vi "DSDLL Digitizing Process.vi"(8 "error in":errorcluster, 11 "dsdll session":variant) -> (0 "error out":errorcluster, 3 "auxiliary data out":variant)   [LabVIEW 2020, in "DSDLL Virtual Digitizer.lvlib"]
doc: "This is called assynchronously! It is process where niScope digitizers digitize samples, then fetching them and returning them via queue to the calling process. It handles both single shot and continuous sampling. For single shot sampling it returns the data in blocks of predifined size after all sampling is done. For streaming mode it streams the data blocks continuously. In any case the calling process must take the data from queue in parallel with this VI otherwise it will overflow! The function also returnes status in the data packet which may be used to determine progess of the digitizing and state of the memory buffer.\nThis VI also returns auxiliary data, i.e. structure with scaling factors, time stamps and measured temperature during sampling."
uses:
  DSDLL Virtual Digitizer.lvlib
  DSDLL Session.ctl
  dsdll/dsdll_instance.ctl
  dsdll/dsdll_device_record.ctl
  DSDLL Process Config.ctl
  DSDLL Data Packet.ctl
  DSDLL Aux Record Data.ctl
  dsdll/dsdll_capture_wave_auto_float32.vi
  dsdll/dsdll.lvlib
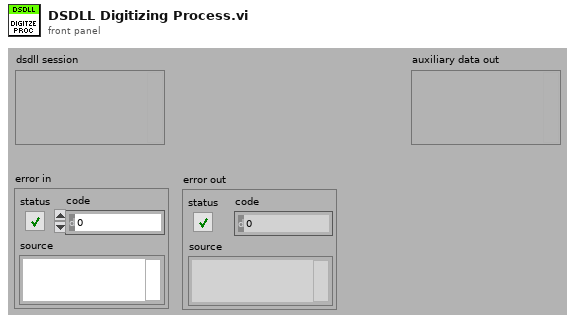
[diagram p1: front panel]
types:
  T1 = typedef "DSDLL Virtual Digitizer.lvlib/DSDLL Session.ctl" = cluster{"dsdll":T2, "channels":i32, "device id":i32, "channel idns":string[], "proc setup":T4, "samples count":i32, "fs [Hz]":dbl}
  T2 = typedef "dsdll.lvlib/dsdll_instance.ctl" = cluster{"dsdll path":path, "dsdll handle":u8[], "output devices":T3[], "capture devices":T3[]}
  T3 = typedef "dsdll.lvlib/dsdll_device_record.ctl" = cluster{"guid":u8[], "name":string}
  T4 = typedef "DSDLL Virtual Digitizer.lvlib/DSDLL Process Config.ctl" = cluster{"packet size [smpl]":i32, "current timeout [s]":dbl, "blk2blk timeout [s]":dbl, "event time":timestamp, "data queue":refnum<queue>, "stop notifier":refnum<notifier>, "proc ref":refnum<vi>}
  T5 = typedef "DSDLL Virtual Digitizer.lvlib/DSDLL Aux Record Data.ctl" = cluster{"time stamp [s]":dbl[], "gain":dbl[], "increment [s]":dbl, "valid?":bool, "abs timestamp":timestamp}
  T6 = typedef "DSDLL Virtual Digitizer.lvlib/DSDLL Data Packet.ctl" = cluster{"int32":i32[][], "card buffer [%]":dbl, "all done?":bool, "offset [smpl]":i32, "sampling?":bool, "queue buffer [%]":dbl, "count [smpl]":i32, "valid?":bool}
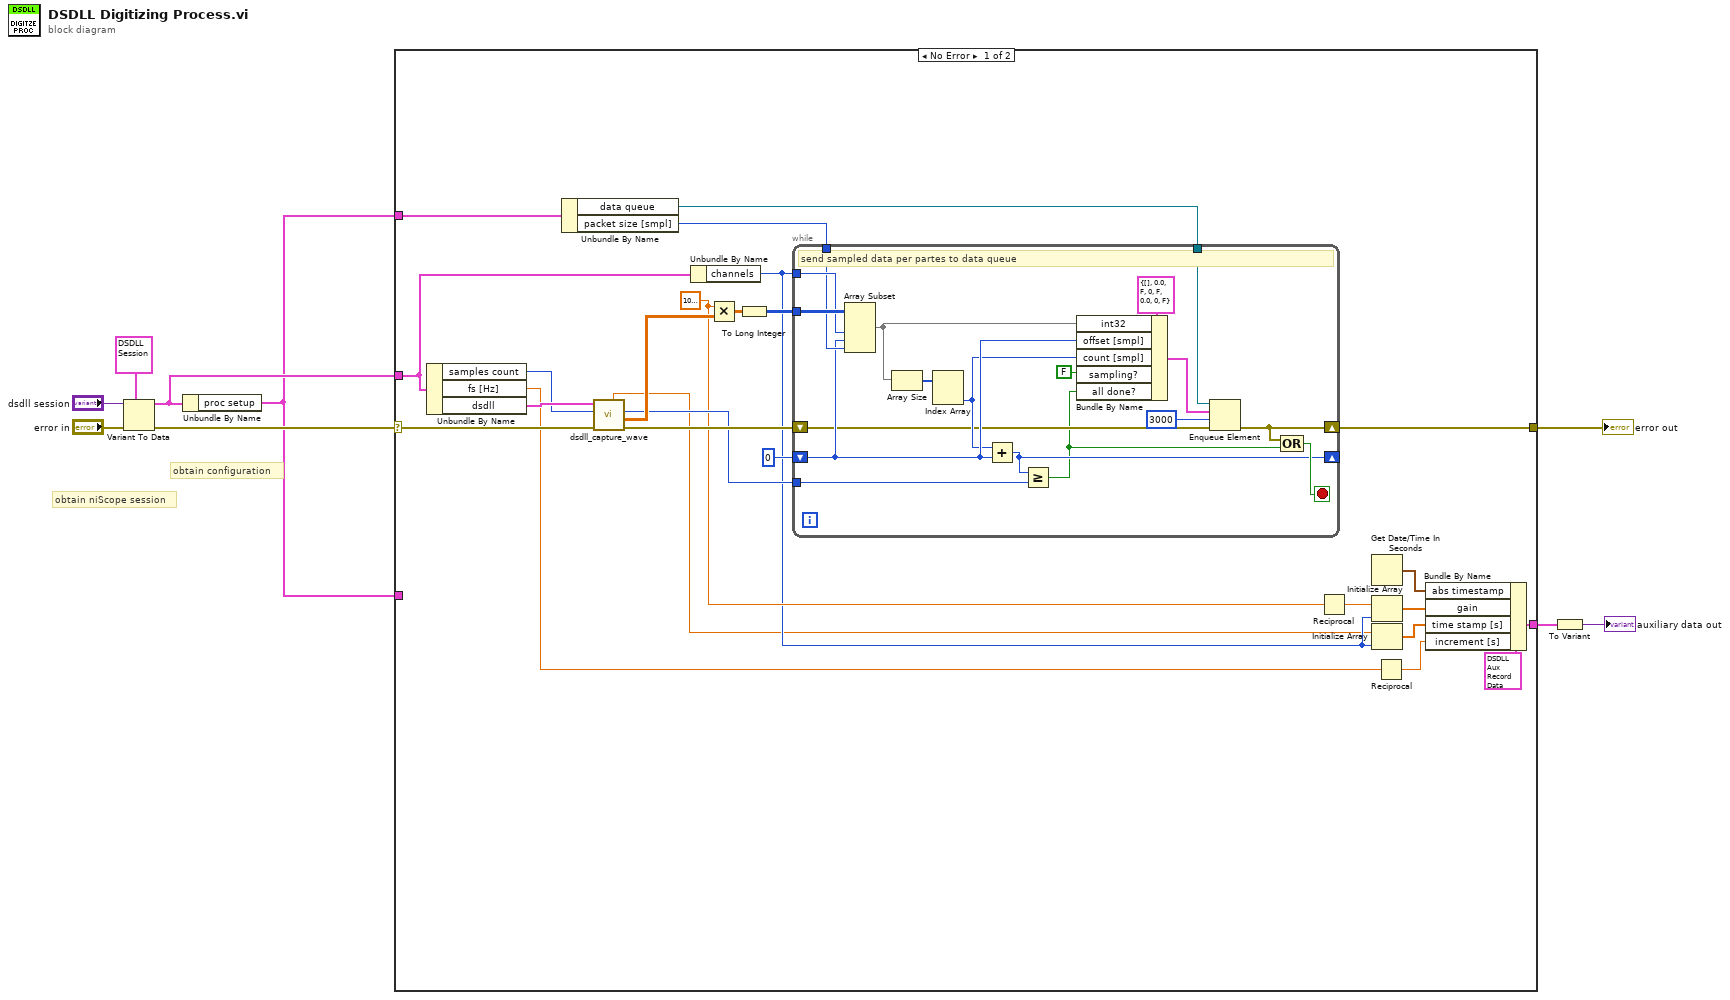
[diagram p0: block diagram]
diagram:
  # "obtain configuration"
  # "obtain niScope session"
  n1 = Variant To Data(error in="error in", type=T1 {"dsdll"={"dsdll path"=path "", "dsdll handle"=[], "output devices"=[], "capture devices"=[]}, "channels"=0, "device id"=0, "channel idns"=[], "proc setup"={"packet size [smpl]"=0, "current timeout [s]"=0.0, "blk2blk timeout [s]"=0.0, "event time"=timestamp(0 s since 1904-01-01), "data queue"=refnum, "stop notifier"=refnum, "proc ref"=refnum}, "samples count"=0, "fs [Hz]"=0.0} ("niScope out"), Variant="dsdll session") -> (data=w3:T1, error out=w2:errorcluster)
  n2 = Unbundle By Name(w3) -> ("proc setup"=w1:T4)
  n3 = case shown="No Error" w2 {
    selector: w2 -> [w34 w53]
    tunnel: w1 -> [_ _]
    tunnel: [w22 w53] -> w4
    tunnel: w3 -> [w27 _]
    tunnel: [w21 _] -> w6
    tunnel: w1 -> [w26 _]
    frame No Error {
      w19 = sgl 1000000000.0
      n4 = Unbundle By Name(w27) -> ("samples count"=w11:i32, "fs [Hz]"=w12:dbl, "dsdll"=w33:T2)
      n5 = Unbundle By Name(w26) -> ("data queue"=w24:refnum<queue>, "packet size [smpl]"=w25:i32)
      n6 = call-poly "dsdll_capture_wave.vi"("error in"=w34, "samples count in"=w11, "dsdll instance in"=w33) -> ("error out"=w32:errorcluster, "float32 waves"=w31:sgl[][], "samples count out"=w23:u32, "time stamp [s]"=w14:dbl)  [unwired: 3 in, 2 out]
      n7 = Unbundle By Name(w27) -> ("channels"=w15:i32)
      n8 = Multiply(x=w19, y=w31) -> (x*y=w30:sgl[][])
      n9 = To Long Integer(number=w30) -> (32bit integer=w29:i32[][])
      n10 = while {
        shift-right: [w39] -> w22
        shift-left: w32 -> [w43]
        tunnel: w29 -> [w52]
        shift-right: [w37] -> _
        shift-left: 0 -> [w46]
        tunnel: w15 -> [w51]
        tunnel: w25 -> [w50]
        tunnel: w24 -> [w42]
        tunnel: w23 -> [w36]
        stop <- w40 stop-if-true
        # "send sampled data per partes to data queue"
        n11 = Array Subset(array=w52, length (row)=w51, index (col)=w46, length (col)=w50) -> (w47:i32[][])  [unwired: 1 in]
        n12 = Array Size(array=w47) -> (size(s)=w49:i32[])
        n13 = Index Array(array=w49) -> (element #2=w45:i32)  [unwired: 2 in, 1 out]
        n14 = Add(x=w45, y=w46) -> (x+y=w37:i32)
        n15 = Greater Or Equal?(x=w37, y=w36) -> (x >= y?=w35:bool)
        n16 = Bundle By Name(cluster=T6 {"int32"=[], "card buffer [%]"=0.0, "all done?"=FALSE, "offset [smpl]"=0, "sampling?"=FALSE, "queue buffer [%]"=0.0, "count [smpl]"=0, "valid?"=FALSE} ("niScope packet"), "int32"=w47, "offset [smpl]"=w46, "count [smpl]"=w45, "sampling?"=FALSE, "all done?"=w35) -> (w38:T6)
        n17 = Enqueue Element(queue=w42, element=w38, timeout in ms (-1)=3000, error in (no error)=w43) -> (error out=w39:errorcluster)  [unwired: 2 out]
        n18 = Compound Arithmetic op=OR(w39, w35) -> (w40:bool)
      }
      n19 = Reciprocal(x=w19) -> (1/x=w17:sgl)
      n20 = Get Date/Time In Seconds() -> (seconds since 1Jan1904=w10:timestamp)
      n21 = Initialize Array(w17, w15) -> (w18:sgl[])
      n22 = Initialize Array(w14, w15) -> (w16:dbl[])
      n23 = Reciprocal(x=w12) -> (1/x=w13:dbl)
      n24 = Bundle By Name(cluster=T5 {"time stamp [s]"=[], "gain"=[], "increment [s]"=0.0, "valid?"=FALSE, "abs timestamp"=timestamp(0 s since 1904-01-01)} ("aux data"), "abs timestamp"=w10, "gain"=w18, "time stamp [s]"=w16, "increment [s]"=w13) -> (w21:T5)
    }
    frame Error {
    }
  }
  "error out" <- w4
  n25 = To Variant(anything=w6) -> (Variant=→"auxiliary data out":variant)
